vi "1D Array (Zeros).vi"(1 "dimension size":i32=1, 4 "value":dbl format="%#_13g") -> (15 "initialized array":dbl[](array[numeric]))   [LabVIEW 2014]
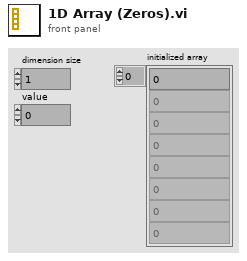
[diagram p1: front panel]
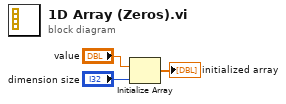
[diagram p0: block diagram]
diagram:
  n1 = Initialize Array("value", "dimension size") -> (→"initialized array":dbl[])
